vi "FindAverageFRF.vi"(4 "Output":u16(ring)=1 items=["Accelerometer", "Accel (speed)", "Microphone", "Vibrometer"], 5 "Method":enum16{"Sqrt(H1H2)", "H1", "H2"}(ring), 6 "delay":dbl, 8 "Microphone Spectrum":cluster{dbl, "df":dbl, "FFT {X}":cdb[]}[](array[cluster]), 11 "Hammer Spectrum":cluster{dbl, "df":dbl, "FFT {X}":cdb[]}[](array[cluster])) -> (0 "Coherence":cluster{"x0":dbl, "df":dbl, dbl[]}(graph), 1 "Complex FRF":cluster{"t0":dbl, "dt":dbl, "Y":cdb[]}, 3 "Average FRF":cluster{"x0":dbl, "df":dbl, dbl[]}(graph))   [LabVIEW 2022 SP3]
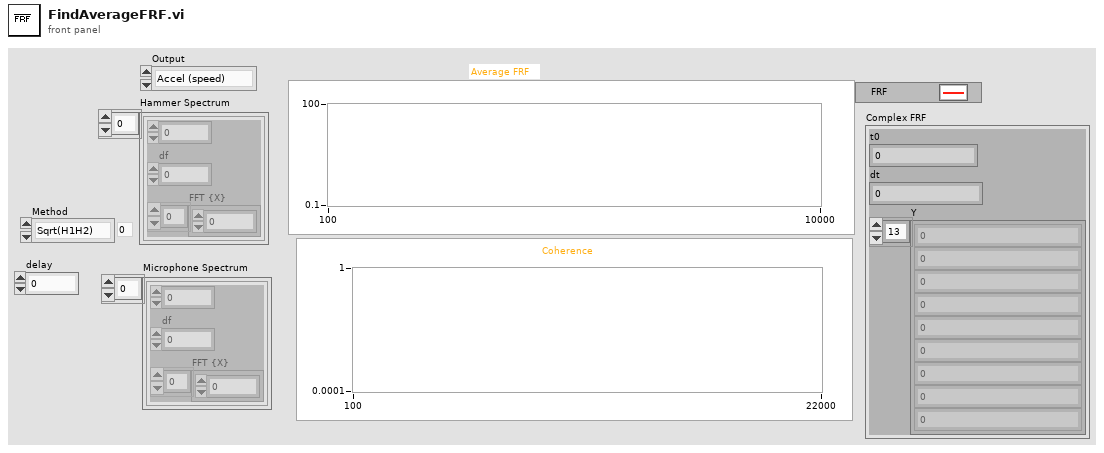
[diagram p1: front panel]
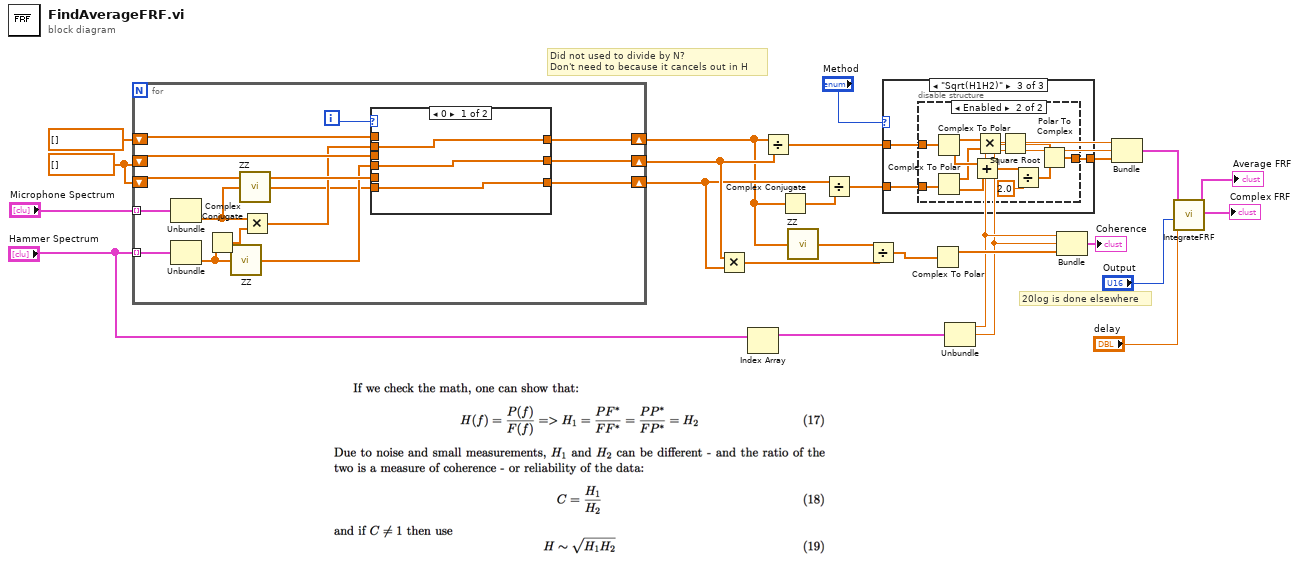
[diagram p0: block diagram]
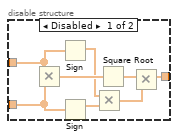
[diagram p4: hidden frame]
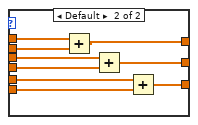
[diagram p5: hidden frame]
diagram:
  w21 = dbl[] [] ("FF*")
  # "20log is done elsewhere"
  # "Did not used to divide by N?\nDon't need to because it cancels out in H"
  n1 = for {
    shift-right: [w39] -> w14
    shift-left: cdb[] [] ("PF*") -> [w40]
    shift-right: [w35] -> w16
    shift-left: w21 -> [w38]
    shift-right: [w36] -> w15
    shift-left: w21 -> [w37]
    tunnel: "Hammer Spectrum" -> [w31] mode=indexing
    tunnel: "Microphone Spectrum" -> [w30] mode=indexing
    i -> [w34]
    n2 = Unbundle(w30) -> ("FFT {X}"=w29:cdb[])  [unwired: 2 out]
    n3 = Unbundle(w31) -> ("FFT {X}"=w33:cdb[])  [unwired: 2 out]
    n4 = Complex Conjugate(1:w33) -> (0:w32:cdb[])
    n5 = call "ZZ.vi"("P"=w33) -> ("PP*"=w27:dbl[])
    n6 = call "ZZ.vi"("P"=w29) -> ("PP*"=w26:dbl[])
    n7 = Multiply(x=w29, y=w32) -> (x*y=w28:cdb[])
    n8 = case shown="0" w34 {
      tunnel: w28 -> [w43 w52]
      tunnel: w40 -> [_ w51]
      tunnel: [w43 w50] -> w39
      tunnel: w38 -> [_ w49]
      tunnel: w37 -> [_ w48]
      tunnel: w26 -> [w41 w47]
      tunnel: [w41 w46] -> w36
      tunnel: w27 -> [w42 w45]
      tunnel: [w42 w44] -> w35
      frame 0 {
      }
      frame Default {
        n9 = Add(x=w51, y=w52) -> (x+y=w50:cdb[])
        n10 = Add(x=w49, y=w45) -> (x+y=w44:dbl[])
        n11 = Add(x=w48, y=w47) -> (x+y=w46:dbl[])
      }
    }
  }
  n12 = Multiply(x=w16, y=w15) -> (x*y=w24:dbl[])
  n13 = Index Array(array="Hammer Spectrum") -> (element=w13:cluster{dbl, "df":dbl, "FFT {X}":cdb[]})  [unwired: 1 in]
  n14 = Divide(x=w14, y=w16) -> (x/y=w10:cdb[])
  n15 = Complex Conjugate(1:w14) -> (0:w17:cdb[])
  n16 = call "ZZ.vi"("P"=w14) -> ("PP*"=w25:dbl[])
  n17 = Divide(x=w15, y=w17) -> (x/y=w11:cdb[])
  n18 = Divide(x=w25, y=w24) -> (x/y=w23:dbl[])
  n19 = case shown="\"Sqrt(H1H2)\"" "Method" {
    tunnel: w11 -> [_ w54 w57]
    tunnel: w10 -> [w53 _ w56]
    tunnel: [w53 w54 w55] -> w6
    frame "H1" {
    }
    frame "H2" {
    }
    frame "Sqrt(H1H2)" {
      n20 = disable-structure shown="Enabled" {
        disable-tunnel: w57 -> [w63 w77]
        disable-tunnel: w56 -> [w64 w76]
        disable-tunnel: [w58 w71] -> w55
        frame Disabled {
          n21 = Multiply(x=w64, y=w63) -> (x*y=w65:cdb[])
          n22 = Sign(1:w64) -> (0:w61:cdb[])
          n23 = Sign(1:w63) -> (0:w62:cdb[])
          n24 = Multiply(x=w61, y=w62) -> (x*y=w59:cdb[])
          n25 = Square Root(x=w65) -> (sqrt(x)=w60:cdb[])
          n26 = Multiply(x=w60, y=w59) -> (x*y=w58:cdb[])
        }
        frame Enabled {
          n27 = Complex To Polar(r * e^(i*theta)=w76) -> (r=w69:dbl[], theta=w75:dbl[])
          n28 = Complex To Polar(r * e^(i*theta)=w77) -> (r=w67:dbl[], theta=w74:dbl[])
          n29 = Add(x=w75, y=w74) -> (x+y=w73:dbl[])
          n30 = Multiply(x=w69, y=w67) -> (x*y=w68:dbl[])
          n31 = Square Root(x=w68) -> (sqrt(x)=w66:dbl[])
          n32 = Divide(x=w73, y=2.0) -> (x/y=w70:dbl[])
          n33 = Polar To Complex(1:w70, 2:w66) -> (0:w71:cdb[])
        }
      }
    }
  }
  n34 = Complex To Polar(r * e^(i*theta)=w23) -> (r=w20:dbl[])  [unwired: 1 out]
  n35 = Unbundle(w13) -> (w3:dbl, "df"=w2:dbl)  [unwired: 1 out]
  n36 = Bundle(w3, "df"=w2, w20) -> (→"Coherence":cluster{dbl, "df":dbl, dbl[]})  [unwired: 1 in]
  n37 = Bundle(w3, "df"=w2, w6) -> (w5:cluster{dbl, "df":dbl, cdb[]})  [unwired: 1 in]
  n38 = call "IntegrateFRF.vi"("delay (sec)"="delay", "Output"="Output", "Complex FRF"=w5) -> ("Complex FRF out"=→"Complex FRF":cluster{"t0":dbl, "dt":dbl, "Y":cdb[]}, "FRF out"=→"Average FRF":cluster{"t0":dbl, "dt":dbl, dbl[]})  [unwired: 7 in]
